vi "Yaw.vi"() -> ()   [LabVIEW 2018]
panel:
  out "Yaw":dbl
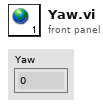
[diagram p1: front panel]
diagram:
